vi "arreglos.vi"() -> ()   [LabVIEW 2020]
panel:
  in  "Array 5":dbl[][](array[numeric])
  out "appended array":dbl[](array[numeric])
  in  "A 6":dbl
  in  "A 5":dbl
  in  "A 4":dbl
  in  "A 3":dbl
  in  "A 2":dbl
  in  "A 1":dbl
  out "Array 4":dbl[](array[numeric])
  in  "Array 3":string[](array[string])
  in  "Array 2":bool[](array[boolean])
  in  "Array":dbl[](array[numeric])
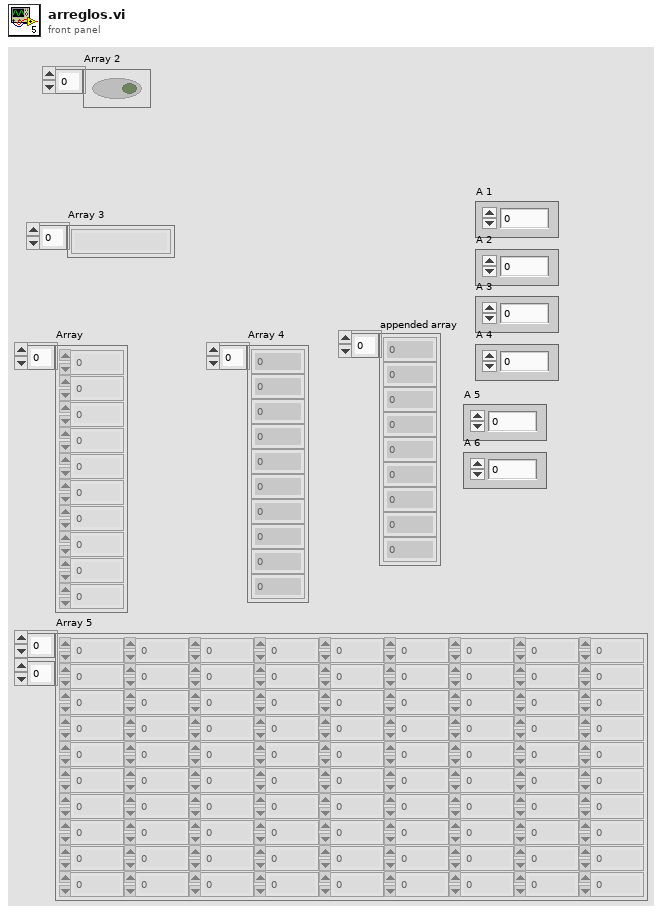
[diagram p1: front panel]
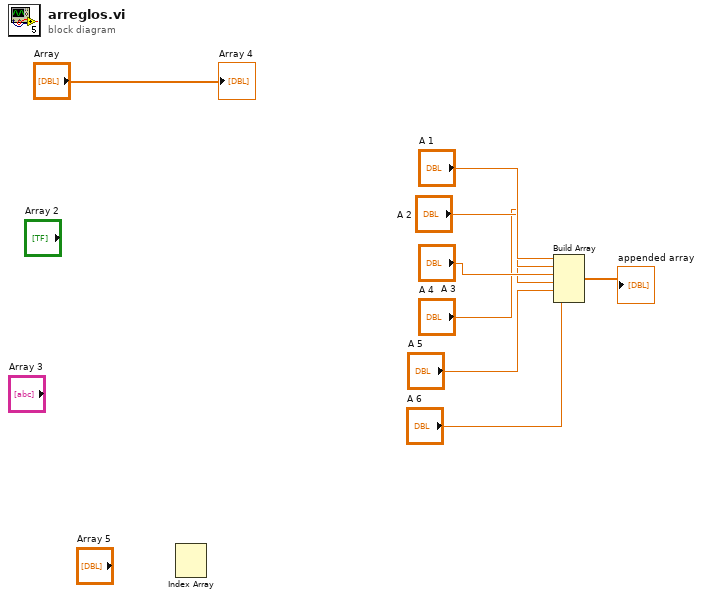
[diagram p0: block diagram]
diagram:
  n1 = Index Array() -> ()  [unwired: 3 in, 2 out]
  n2 = Build Array("A 1", "A 2", "A 3", "A 4", "A 5", "A 6") -> (→"appended array":dbl[])
  "Array 4" <- "Array"
